vi "UDP ESSENTIAL SENDER.vi"(7 "milliseconds to wait (LoopTimer)":u32, 8 "error in (no error)":errorcluster, 9 "destination adress":string, 10 "destination port":u16, 11 "UDP Network Connection in":refnum<k16>) -> (0 "error out":errorcluster)   [LabVIEW 2016]
uses:
  Globale Variablen VI/Global Variables.vi
  Globale Variablen VI/RadSensoren.vi
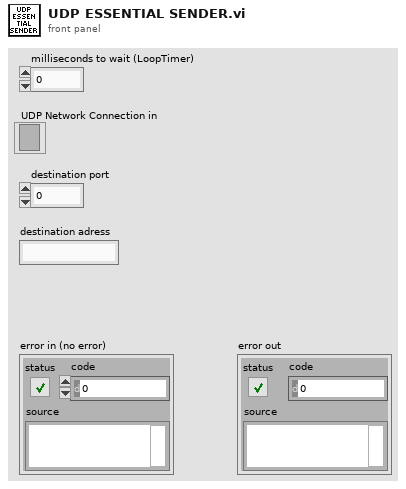
[diagram p1: front panel]
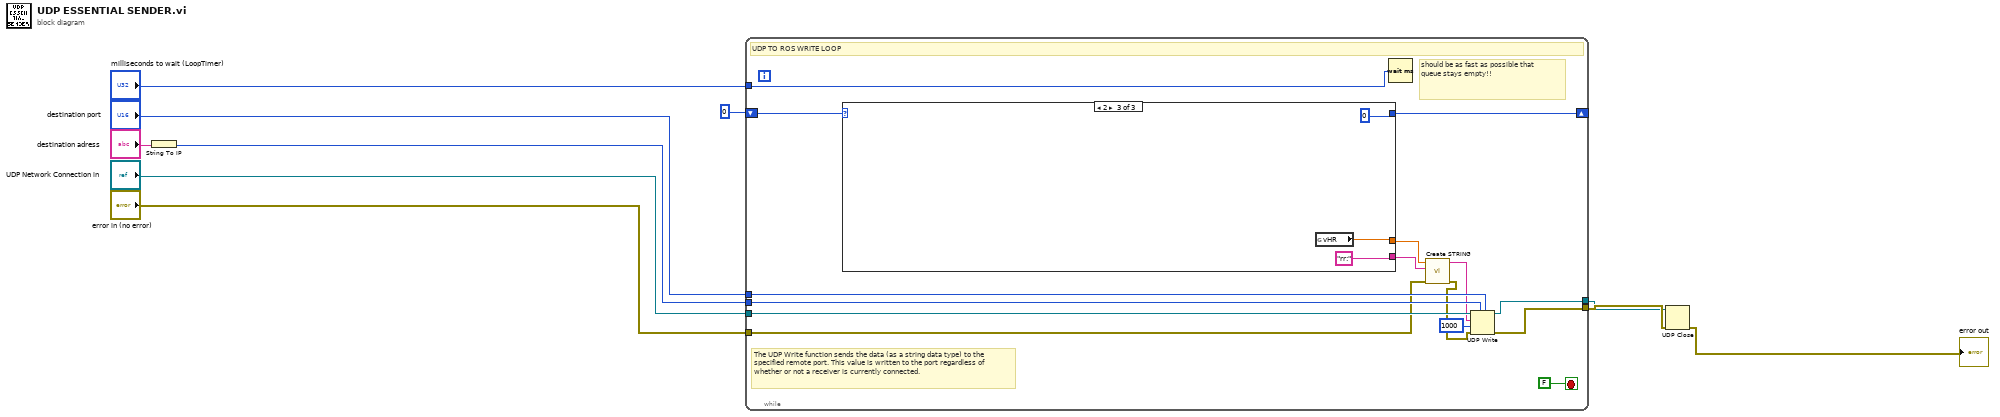
[diagram p0: block diagram]
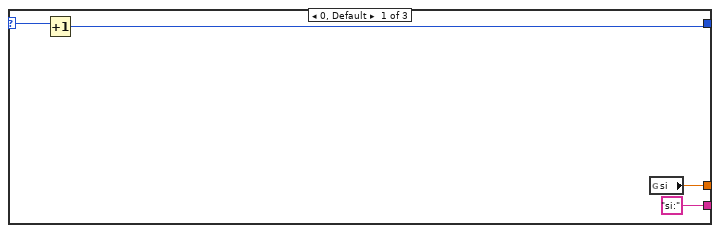
[diagram p2: hidden frame]
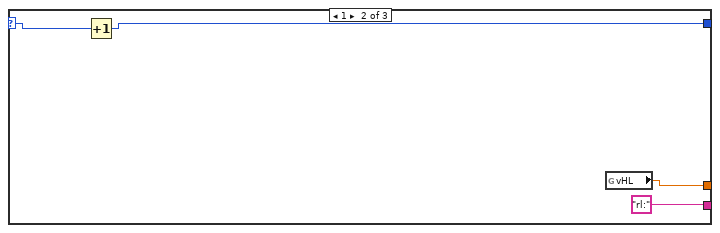
[diagram p3: hidden frame]
diagram:
  n1 = String To IP(1:"destination adress") -> (0:w7:u32)
  n2 = while {
    tunnel: [w12] -> w9
    tunnel: "destination port" -> [w25]
    tunnel: w7 -> [w24]
    tunnel: "UDP Network Connection in" -> [w23]
    tunnel: "error in (no error)" -> [w15]
    tunnel: [w22] -> w8
    tunnel: "milliseconds to wait (LoopTimer)" -> [w21]
    shift-right: [w19] -> _
    shift-left: 0 -> [w18]
    stop <- FALSE stop-if-true
    # "should be as fast as possible that queue stays empty!!"
    # "The UDP Write function sends the data (as a string data type) to the specified remote port. This value is written to the port regardless of whether or not a receiver is currently connected."
    # "UDP TO ROS WRITE LOOP"
    n3 = case shown="2" w18 {
      selector: w18 -> [w27 w31 _]
      tunnel: [w26 w30 0] -> w19
      tunnel: [w29 w33 w36] -> w17
      tunnel: ["si:" "rl:" "rr:"] -> w16
      frame 0, Default {
        n4 = Increment(x=w27) -> (x+1=w26:i32)
        n5 = global read "Global Variables.vi" "si"() -> (w29:dbl)
      }
      frame 1 {
        n6 = Increment(x=w31) -> (x+1=w30:i32)
        n7 = global read "RadSensoren.vi" "vHL"() -> (w33:sgl)
      }
      frame 2 {
        n8 = global read "RadSensoren.vi" "vHR"() -> (w36:sgl)
      }
    }
    n9 = Wait (ms)(milliseconds to wait=w21) -> ()  [unwired: 1 out]
    n10 = call "Create STRING.vi"("error in (no error)"=w15, "Descriptor"=w16, "Value IN"=w17) -> ("error out"=w14:errorcluster, "concatenated string"=w13:string)  [unwired: 7 in]
    n11 = UDP Write(address=w24, port or service name=w25, connection ID=w23, data in=w13, 8:w14, 9:1000 ("timeout ms (25000)")) -> (error out=w12:errorcluster, 3:w22:refnum<k16>)
  }
  n12 = UDP Close(connection ID=w8, 8:w9) -> (error out=→"error out":errorcluster)  [unwired: 1 out]
